vi "fire error event.vi"(8 "Error to Process":errorcluster, 9 "Report Error (F)":bool, 10 "Severity (Do Nothing)":T1=enum."Do Nothing", 11 "Error Source":refnum<class "Template.lvclass">) -> ()   [LabVIEW 2020, in "Template.lvlib" / "Template.lvclass"]
uses:
  Template.lvclass
  interfaces/Error Interface/Error/typedefs/error severity.ctl
  Template.lvclass/Template.ctl
  interfaces/Error Interface/Error/Error.lvclass
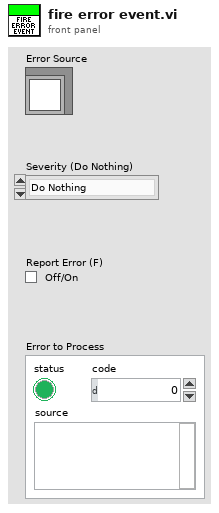
[diagram p1: front panel]
types:
  T1 = typedef "Error Interface.lvlib/Error.lvclass/error severity.ctl" = enum16{"Shutdown", "Restart Calling Actor", "Restart Nested Actor", "Do Nothing"}
  T2 = typedef "Template.lvlib/Template.lvclass/base actor events.ctl" = cluster{"Stop Actor":refnum<user-event>, "New Error":refnum<user-event>, "New Settings":refnum<user-event>}
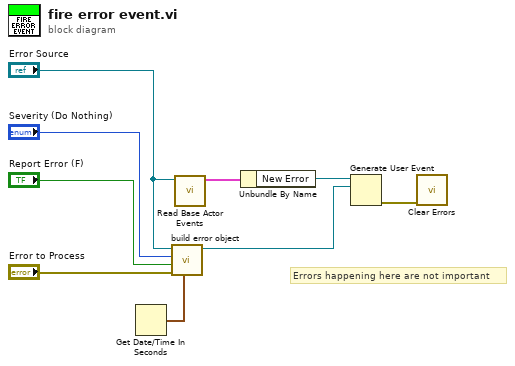
[diagram p0: block diagram]
diagram:
  # "Errors happening here are not important"
  n1 = Get Date/Time In Seconds() -> (seconds since 1Jan1904=w2:timestamp)
  n2 = call "build error object.vi"("Time Stamp"=w2, "Error to Process"="Error to Process", "Report Error (F)"="Report Error (F)", "Severity (Do Nothing)"="Severity (Do Nothing)", "Error Location"="Error Source") -> ("Error object"=w7:refnum<class "Error.lvclass">)  [unwired: 6 in]
  n3 = call "Read Base Actor Events.vi"("Template in"="Error Source") -> ("Base Actor Events"=w3:T2)  [unwired: 10 in]
  n4 = Unbundle By Name(w3) -> ("New Error"=w6:refnum<user-event>)
  n5 = Generate User Event(user event=w6, event data cluster=w7) -> (error out=w1:errorcluster)  [unwired: 2 in, 1 out]
  n6 = call <vilib>:"Clear Errors.vi"("error in (no error)"=w1) -> ()  [unwired: 5 in, 2 out]
